vi "Proiect_senzori.vi"() -> ()   [LabVIEW 2024]
panel:
  out "Panou de control lumini":string
  in  "Lumina aprinsa garaj":bool
  in  "Lumina aprinsa debara":bool
  in  "Lumina aprinsa living":bool
  in  "Lumina aprinsa bucatarie":bool
  in  "Lumina aprinsa baie":bool
  in  "Lumina aprinsa hol":bool
  in  "Lumina aprinsa dormitor3":bool
  in  "Lumina aprinsa dormitor2":bool
  in  "Lumina aprinsa dormitor1":bool
  in  "Starea ventilatorului":bool
  in  "Min 2":dbl=18.0
  in  "Max 2":dbl=25.0
  out "?":string
  in  "Control umiditate":dbl(slide) scale=0.0..10.0
  in  "Temperatura":dbl(slide) scale=-20.0..60.0
  in  "a":bool
  out "Alarma":string
  out "Control geamuri":string
  out "?":string
  in  "Min":dbl=18.0
  in  "Max":dbl=25.0
  out "Securitate usa de la intrare":string
  in  "Introdu parola":dbl
  out "?":bool
  out "?":bool
  out "?":bool
  out "?":bool
  out "?":bool
  out "?":bool
  out "?":bool
  out "?":bool
  out "?":bool
  out "?":bool
  in  "Nivel luminã solarã":dbl(slide) scale=0.0..100.0
  out "Putere generata [W]":dbl(slide) scale=0.0..5000.0 scale format="%.2f"
  out "Control usi":string
  in  "Usa de la garaj":bool
  in  "Usa de la baie":bool
  in  "Usa de la dormitor 2":bool
  in  "Usa de la dormitor 3":bool
  in  "Usa de la dormitor 1":bool
  in  "Usa de la bucatarie":bool
  in  "Usa de la debara":bool
  in  "Usa de la living la garaj":bool
  in  "Usa de la living":bool
  in  "Usa de la intrare":bool
  in  "Senzor geam garaj":bool
  in  "Senzor de miscare  garaj":bool
  in  "Geam garaj":bool
  in  "Geam baie":bool
  in  "Geam dormitor3":bool
  in  "Geam dormitor2":bool
  in  "Geam dormitor1":bool
  in  "Geam debara":bool
  in  "Geam bucatarie 1":bool
  in  "Geam bucatarie 2":bool
  in  "Geam living 3":bool
  in  "Geam living 2":bool
  in  "Geam living 1":bool
  in  "Senzor de miscare  living":bool
  in  "Senzor geam living3":bool
  in  "Senzor geam living2":bool
  in  "Senzor geam living1":bool
  in  "Senzor geam dormitor3":bool
  in  "Senzor geam dormitor2":bool
  in  "Senzor geam baie":bool
  in  "Senzor geam dormitor1":bool
  in  "Senzor geam debara":bool
  in  "Senzor geam bucatarie2":bool
  in  "Senzor geam bucatarie1":bool
  in  "Senzor de miscare  baie":bool
  in  "Senzor de miscare dormitor3":bool
  in  "Senzor de miscare dormitor2":bool
  in  "Senzor de miscare dormitor1":bool
  in  "Senzor de miscare debara":bool
  in  "Senzor de miscare bucatarie":bool
  in  "Senzor de miscare hol":bool
  in  "stop":bool
  # "Planul casei inteligente"
  # "Bucatarie"
  # "Dormitor 1"
  # "Debara"
  # "Living"
  # "Hol"
  # "Garaj"
  # "Dormitor 3"
  # "Dormitor 2"
  # "Baie"
  # "Panou fotovoltaic"
  # "Reglare temperatura"
  # "Reglare umiditate"
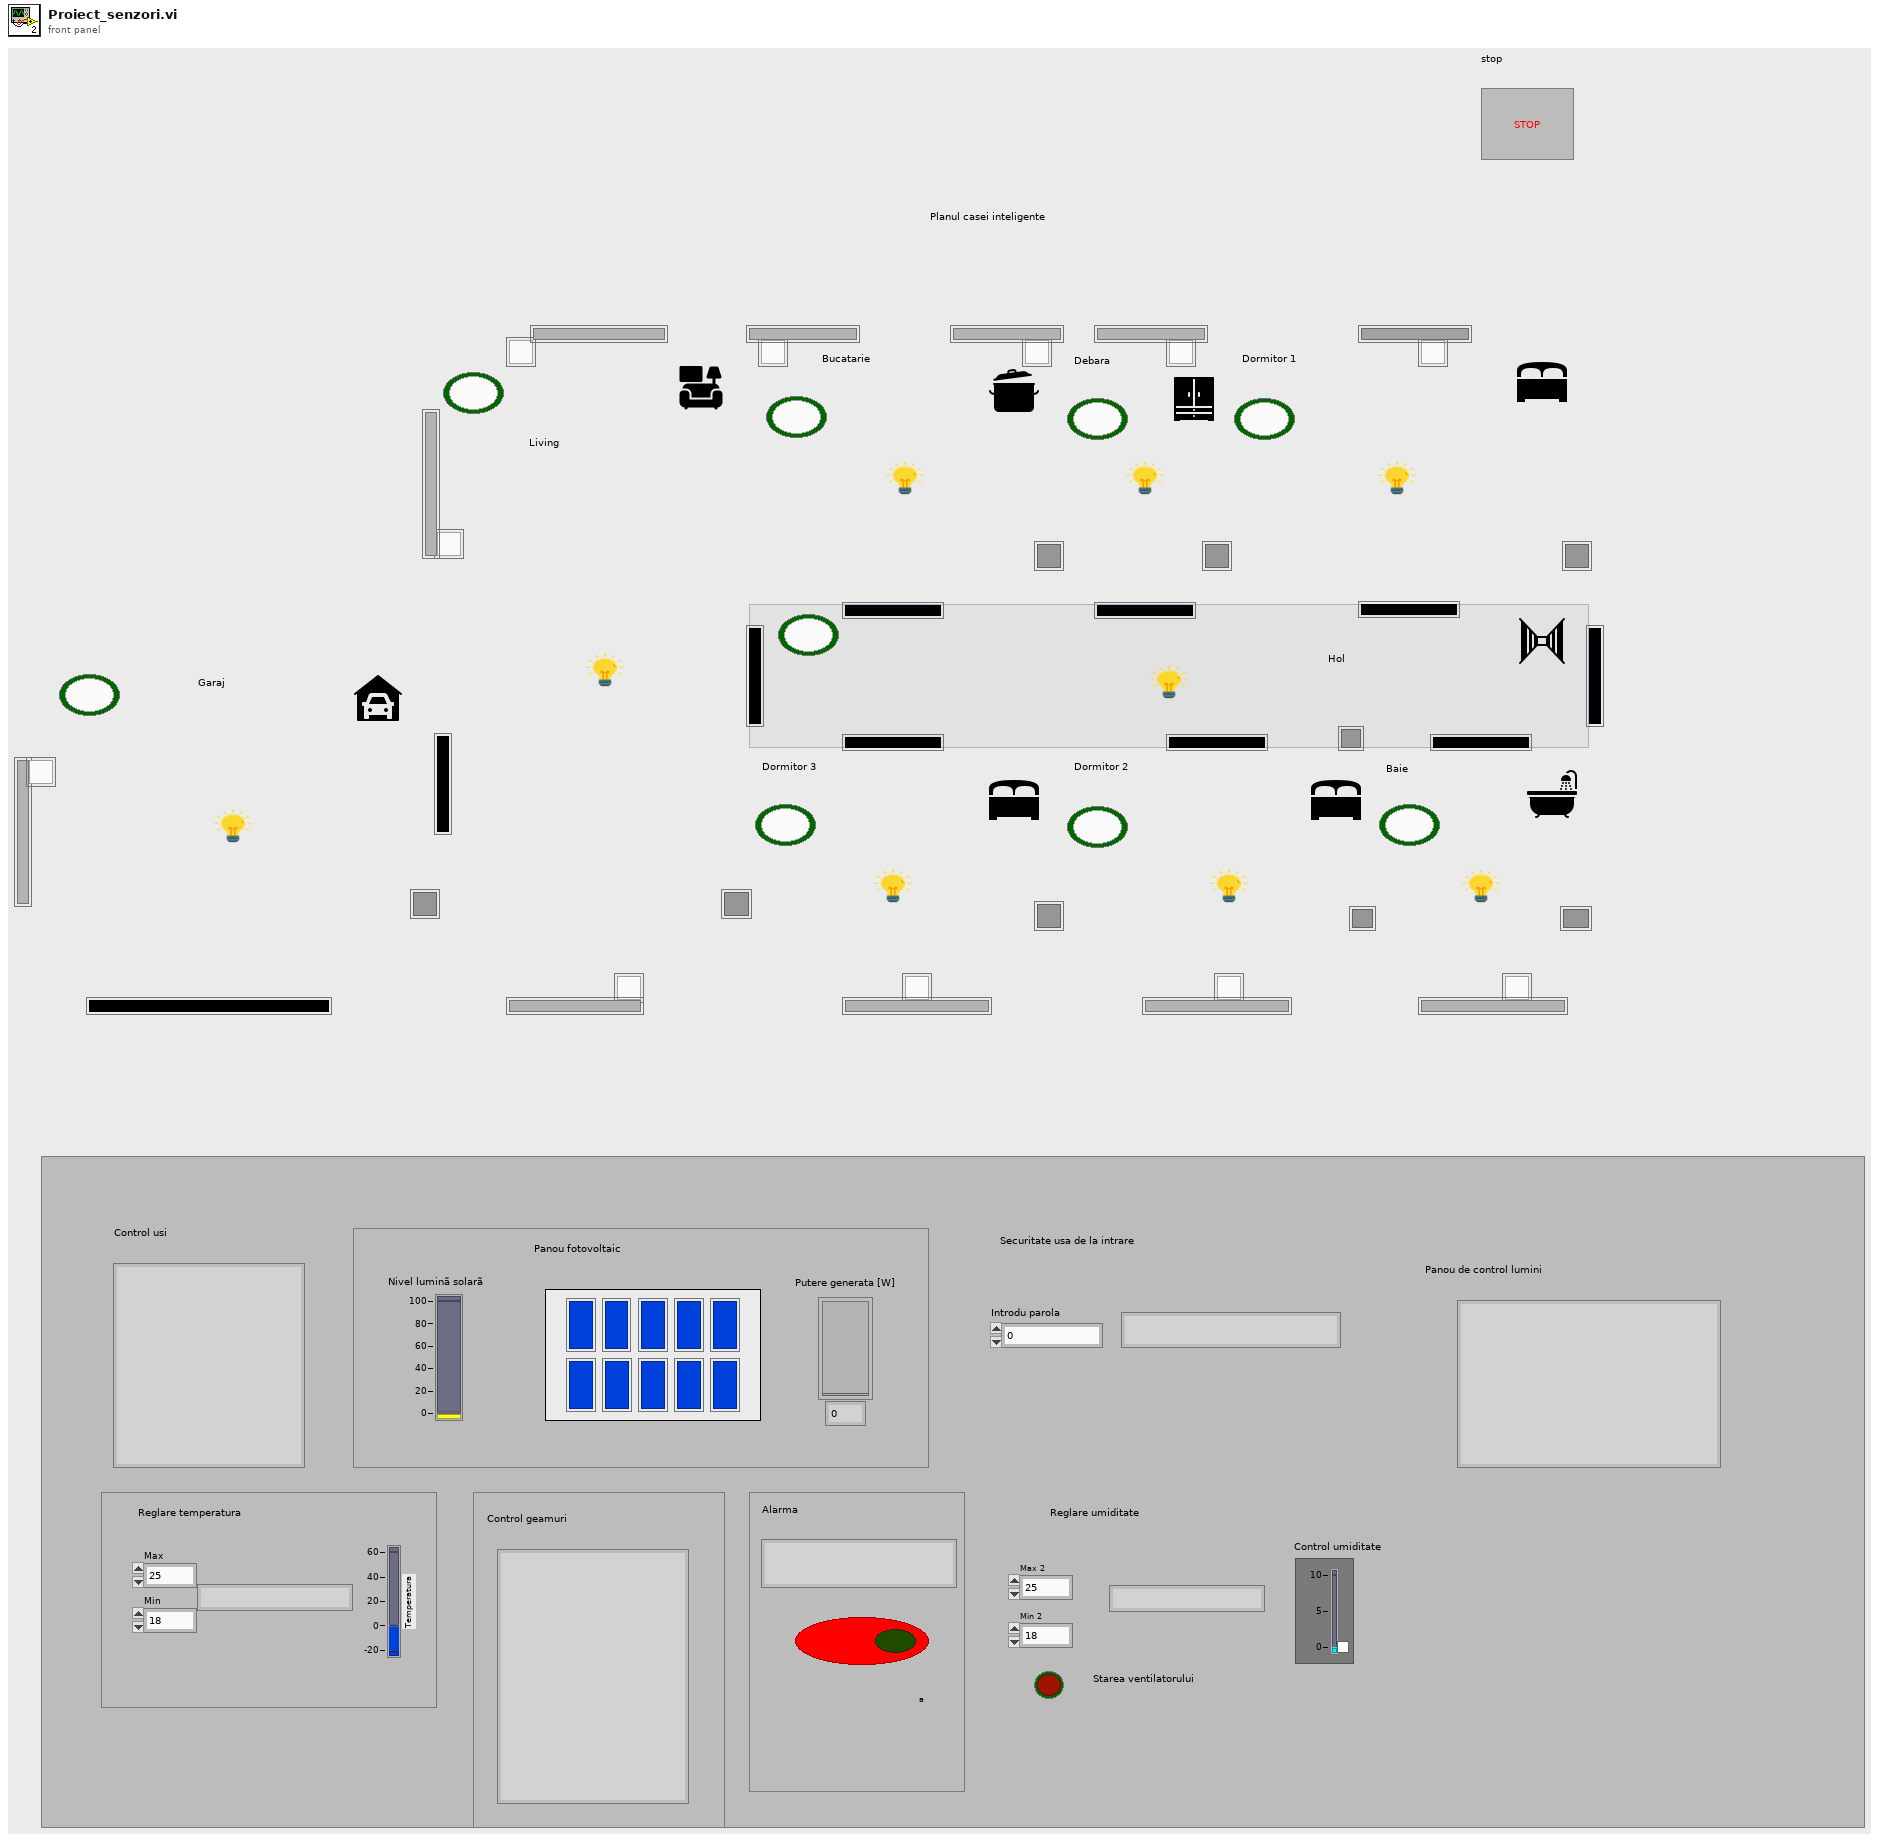
[diagram p1: front panel]
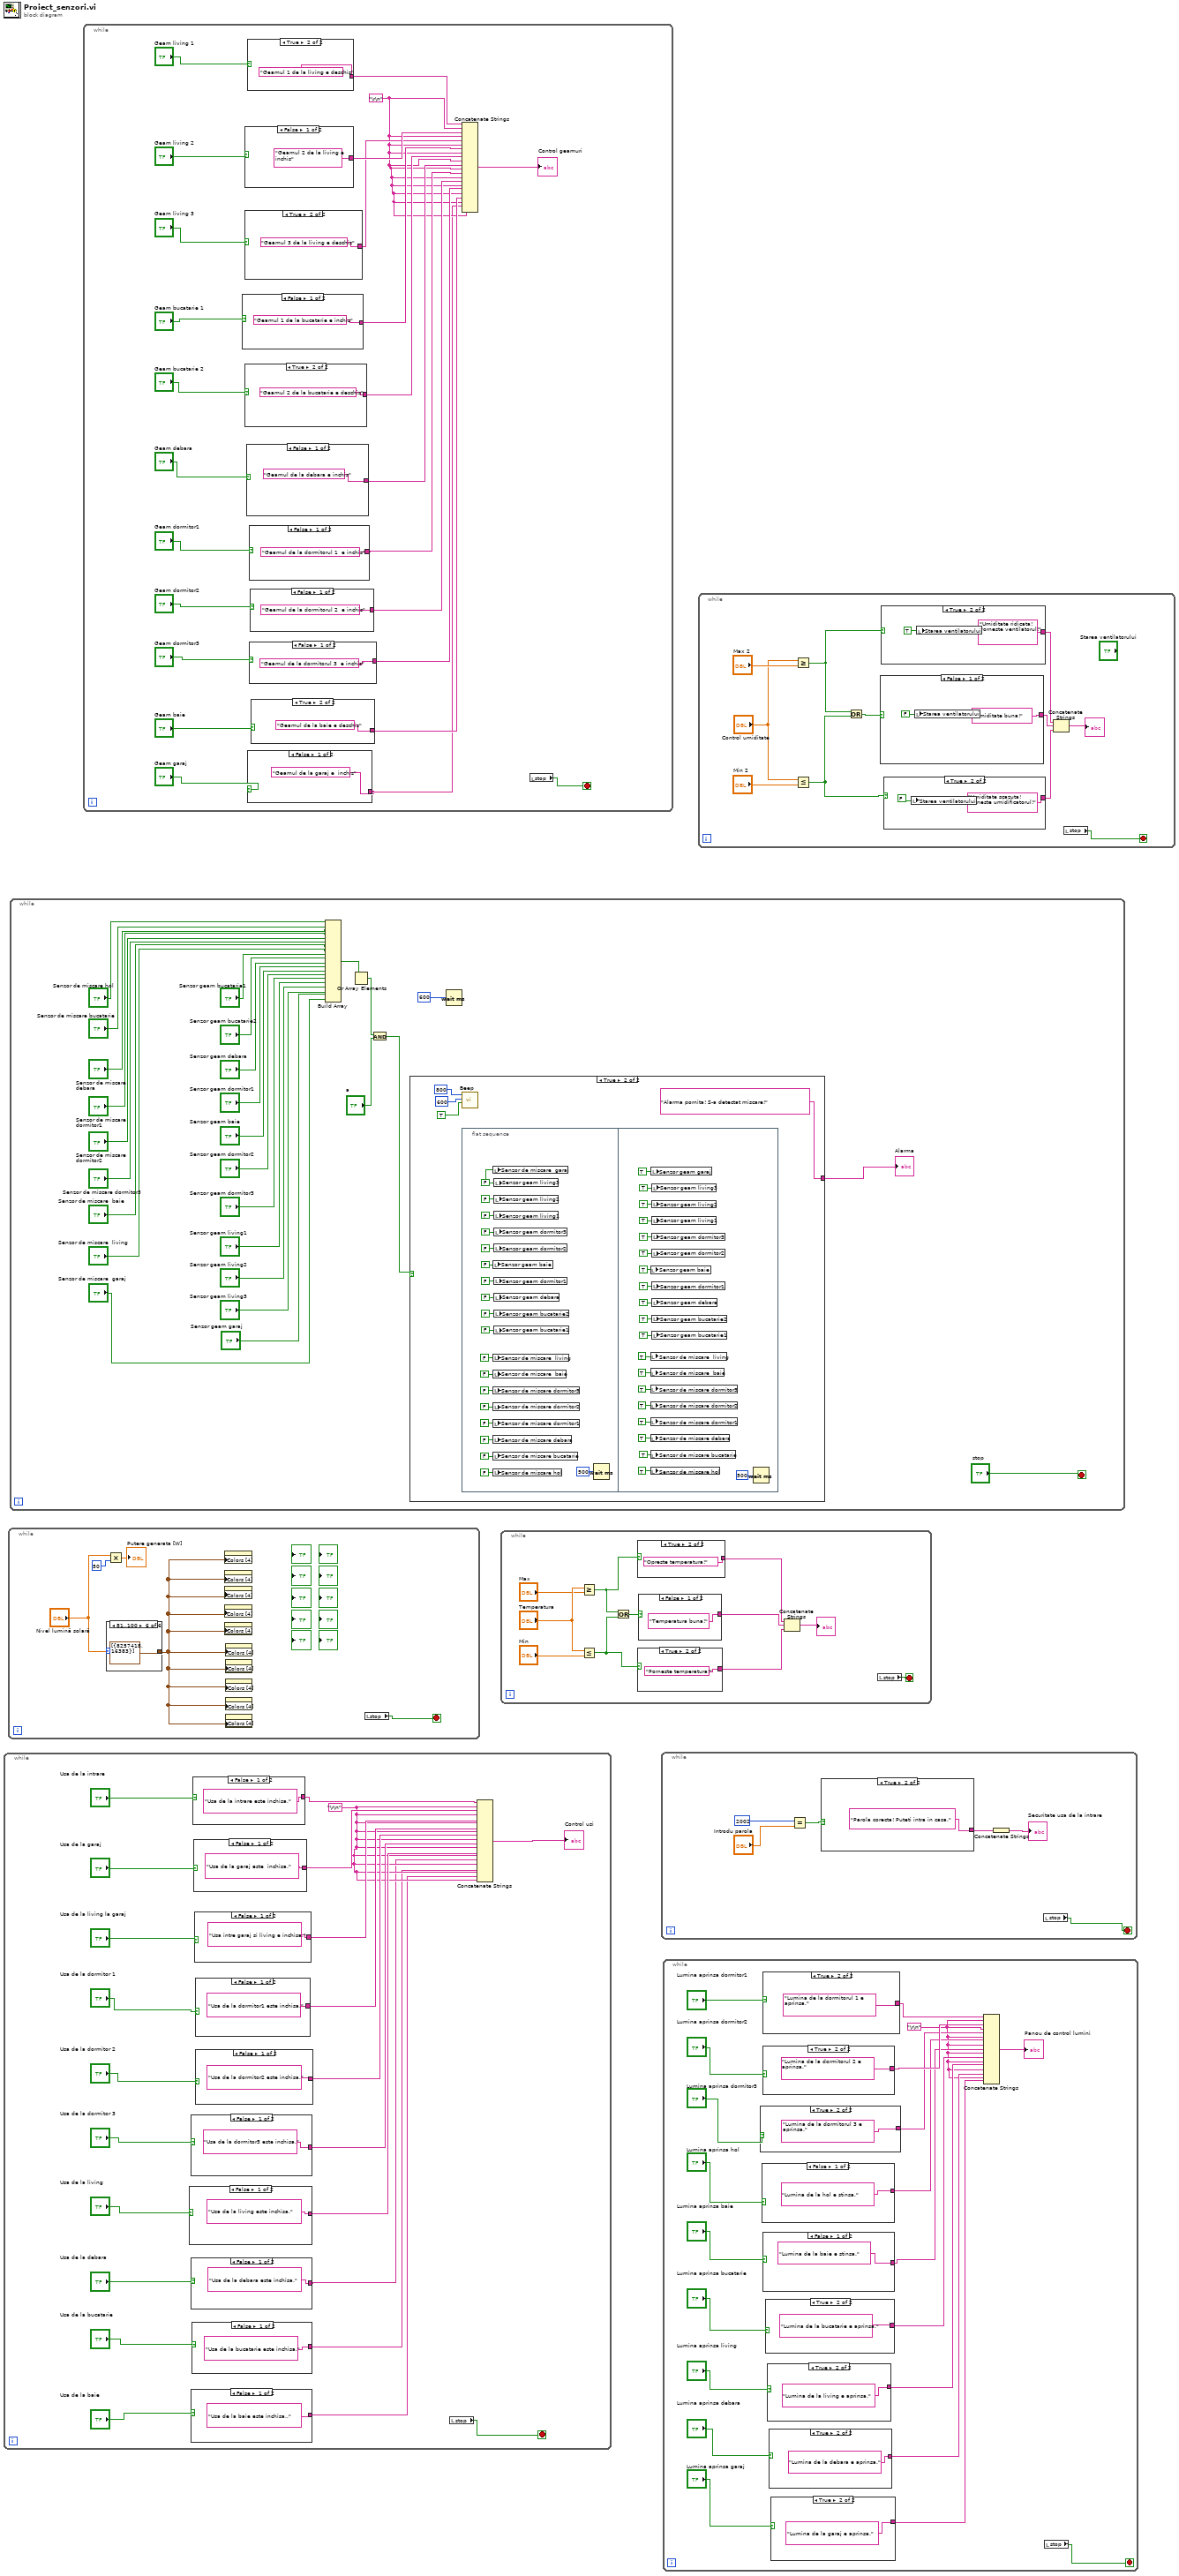
[diagram p0: block diagram]
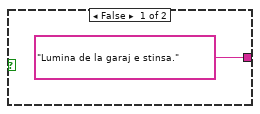
[diagram p2: hidden frame]
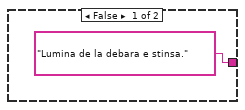
[diagram p3: hidden frame]
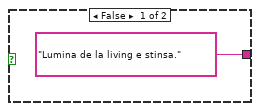
[diagram p4: hidden frame]
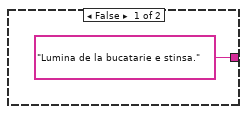
[diagram p5: hidden frame]
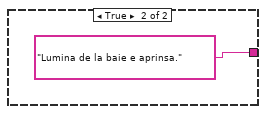
[diagram p6: hidden frame]
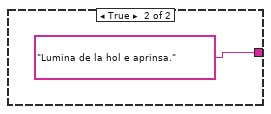
[diagram p7: hidden frame]
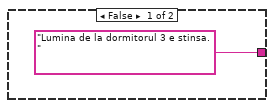
[diagram p8: hidden frame]
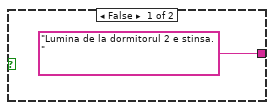
[diagram p9: hidden frame]
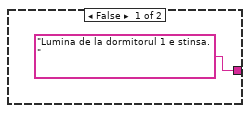
[diagram p10: hidden frame]
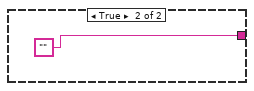
[diagram p11: hidden frame]
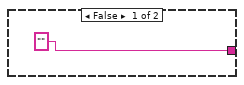
[diagram p12: hidden frame]
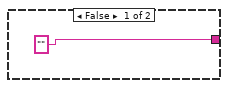
[diagram p13: hidden frame]
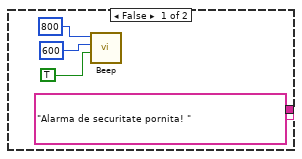
[diagram p14: hidden frame]
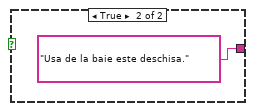
[diagram p15: hidden frame]
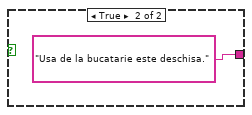
[diagram p16: hidden frame]
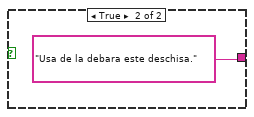
[diagram p17: hidden frame]
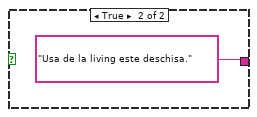
[diagram p18: hidden frame]
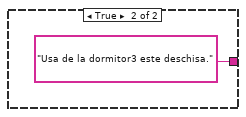
[diagram p19: hidden frame]
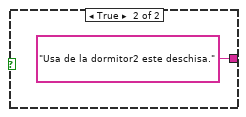
[diagram p20: hidden frame]
diagram:
  n1 = while {
    stop <- w1 stop-if-true
    w6 = "\r\n" ("End of Line Constant")
    n2 = case shown="False" "Usa de la living" {
      tunnel: ["Usa de la living este inchisa." "Usa de la living este deschisa."] -> w7
      frame False {
      }
      frame True {
      }
    }
    n3 = case shown="False" "Usa de la debara" {
      tunnel: ["Usa de la debara este inchisa." "Usa de la debara este deschisa."] -> w5
      frame False {
      }
      frame True {
      }
    }
    n4 = case shown="False" "Usa de la dormitor 3" {
      tunnel: ["Usa de la dormitor3 este inchisa." "Usa de la dormitor3 este deschisa."] -> w8
      frame False {
      }
      frame True {
      }
    }
    n5 = case shown="False" "Usa de la baie" {
      tunnel: ["Usa de la baie este inchisa.." "Usa de la baie este deschisa."] -> w3
      frame False {
      }
      frame True {
      }
    }
    n6 = case shown="False" "Usa de la bucatarie" {
      tunnel: ["Usa de la bucatarie este inchisa." "Usa de la bucatarie este deschisa."] -> w4
      frame False {
      }
      frame True {
      }
    }
    n7 = case shown="False" "Usa de la intrare" {
      tunnel: ["Usa de la intrare este inchisa," "Usa de la intrare este deschisa."] -> w13
      frame False {
      }
      frame True {
      }
    }
    n8 = case shown="False" "Usa de la garaj" {
      tunnel: ["Usa de la garaj este  inchisa." "Usa de la garaj este  deschisa."] -> w12
      frame False {
      }
      frame True {
      }
    }
    n9 = case shown="False" "Usa de la living la garaj" {
      tunnel: ["Usa intre garaj si living e inchisa." "Usa intre garaj si living e deschisa."] -> w11
      frame False {
      }
      frame True {
      }
    }
    n10 = case shown="False" "Usa de la dormitor 1" {
      tunnel: ["Usa de la dormitor1 este inchisa." "Usa de la dormitor1 este deschisa."] -> w10
      frame False {
      }
      frame True {
      }
    }
    n11 = case shown="False" "Usa de la dormitor 2" {
      tunnel: ["Usa de la dormitor2 este inchisa." "Usa de la dormitor2 este deschisa."] -> w9
      frame False {
      }
      frame True {
      }
    }
    n12 = local read "stop"() -> (w1:bool)
    n13 = Concatenate Strings(w13, w6, w12, w6, w11, w6, w10, w6, w9, w6, w8, w6, w7, w6, w5, w6, w4, w6, w3, w6) -> (→"Control usi":string)
  }
  n14 = while {
    stop <- w44 stop-if-true
    n15 = case shown="81..100" "Nivel luminã solarã" {
      tunnel: [cluster{u32, u32}[] [{16860, 16860}] ("Colors [4]") cluster{u32, u32}[] [{15366, 16383}] ("Colors [4]") cluster{u32, u32}[] [{42000, 16383}] ("Colors [4]") cluster{u32, u32}[] [{56598, 16383}] ("Colors [4]") cluster{u32, u32}[] [{2293560, 16383}] ("Colors [4]") cluster{u32, u32}[] [{8257418, 16383}] ("Colors [4]")] -> w45
      frame 0, Default {
      }
      frame 1..20 {
      }
      frame 21..40 {
      }
      frame 41..60 {
      }
      frame 61..80 {
      }
      frame 81..100 {
      }
    }
    n16 = Multiply(x="Nivel luminã solarã", y=50) -> (x*y=→"Putere generata [W]":dbl)
    n17 = property class="Bool (strict)"("Colors [4]"=w45) -> ()  [unwired: 2 in, 2 out]
    n18 = property class="Bool (strict)"("Colors [4]"=w45) -> ()  [unwired: 2 in, 2 out]
    n19 = property class="Bool (strict)"("Colors [4]"=w45) -> ()  [unwired: 2 in, 2 out]
    n20 = property class="Bool (strict)"("Colors [4]"=w45) -> ()  [unwired: 2 in, 2 out]
    n21 = property class="Bool (strict)"("Colors [4]"=w45) -> ()  [unwired: 2 in, 2 out]
    n22 = property class="Bool (strict)"("Colors [4]"=w45) -> ()  [unwired: 2 in, 2 out]
    n23 = property class="Bool (strict)"("Colors [4]"=w45) -> ()  [unwired: 2 in, 2 out]
    n24 = property class="Bool (strict)"("Colors [4]"=w45) -> ()  [unwired: 2 in, 2 out]
    n25 = property class="Bool (strict)"("Colors [4]"=w45) -> ()  [unwired: 2 in, 2 out]
    n26 = property class="Bool (strict)"("Colors [4]"=w45) -> ()  [unwired: 2 in, 2 out]
    n27 = local read "stop"() -> (w44:bool)
  }
  n28 = while {
    stop <- "stop" stop-if-true
    n29 = Build Array "Build Array"("Senzor de miscare hol", "Senzor de miscare bucatarie", "Senzor de miscare debara", "Senzor de miscare dormitor1", "Senzor de miscare dormitor2", "Senzor de miscare dormitor3", "Senzor de miscare  baie", "Senzor de miscare  living", "Senzor geam bucatarie1", "Senzor geam bucatarie2", "Senzor geam debara", "Senzor geam dormitor1", "Senzor geam baie", "Senzor geam dormitor2", "Senzor geam dormitor3", "Senzor geam living1", "Senzor geam living2", "Senzor geam living3", "Senzor geam garaj", "Senzor de miscare  garaj") -> (w80:bool[])
    n30 = Or Array Elements(Boolean array=w80) -> (logical OR=w58:bool)
    n31 = And(x=w58, y="a") -> (x .and. y?=w56:bool)
    n32 = case shown="True" w56 {
      tunnel: ["Alarma oprita! Nu avem niciun pericol. " "Alarma pornita! S-a detectat miscare!"] -> w61
      frame False {
      }
      frame True {
        n33 = call <vilib>:"Beep.vi"("use system alert? (T)"=TRUE, "duration (msec)"=600, "frequency (Hz)"=800) -> ()  [unwired: 9 in]
        n34 = flat-sequence {
          frame #0 {
            w87 = FALSE ("Senzor geam living3")
            n35 = local write "Senzor de miscare  garaj"(w87) -> ()
            n36 = local write "Senzor geam baie"(FALSE ("Senzor geam baie")) -> ()
            n37 = local write "Senzor de miscare  living"(FALSE ("Senzor de miscare  living")) -> ()
            n38 = local write "Senzor de miscare  baie"(FALSE ("Senzor de miscare  baie")) -> ()
            n39 = local write "Senzor de miscare dormitor3"(FALSE ("Senzor de miscare dormitor3")) -> ()
            n40 = local write "Senzor de miscare dormitor2"(FALSE ("Senzor de miscare dormitor2")) -> ()
            n41 = local write "Senzor de miscare dormitor1"(FALSE ("Senzor de miscare dormitor1")) -> ()
            n42 = local write "Senzor de miscare debara"(FALSE ("Senzor de miscare debara")) -> ()
            n43 = local write "Senzor de miscare bucatarie"(FALSE ("Senzor de miscare bucatarie")) -> ()
            n44 = local write "Senzor de miscare hol"(FALSE ("Senzor de miscare hol")) -> ()
            n45 = local write "Senzor geam living3"(w87) -> ()
            n46 = local write "Senzor geam living2"(FALSE ("Senzor geam living2")) -> ()
            n47 = local write "Senzor geam living1"(FALSE ("Senzor geam living1")) -> ()
            n48 = local write "Senzor geam dormitor3"(FALSE ("Senzor geam dormitor3")) -> ()
            n49 = local write "Senzor geam dormitor2"(FALSE ("Senzor geam dormitor2")) -> ()
            n50 = local write "Senzor geam dormitor1"(FALSE ("Senzor geam dormitor1")) -> ()
            n51 = local write "Senzor geam debara"(FALSE ("Senzor geam debara")) -> ()
            n52 = local write "Senzor geam bucatarie2"(FALSE ("Senzor geam bucatarie2")) -> ()
            n53 = local write "Senzor geam bucatarie1"(FALSE ("Senzor geam bucatarie1")) -> ()
            n54 = Wait (ms)(milliseconds to wait=u32 500) -> ()  [unwired: 1 out]
          }
          frame #1 {
            n55 = local write "Senzor geam baie"(TRUE ("Senzor geam baie")) -> ()
            n56 = local write "Senzor de miscare  living"(TRUE ("Senzor de miscare  living")) -> ()
            n57 = local write "Senzor de miscare  baie"(TRUE ("Senzor de miscare  baie")) -> ()
            n58 = local write "Senzor de miscare dormitor3"(TRUE ("Senzor de miscare dormitor3")) -> ()
            n59 = local write "Senzor de miscare dormitor2"(TRUE ("Senzor de miscare dormitor2")) -> ()
            n60 = local write "Senzor de miscare dormitor1"(TRUE ("Senzor de miscare dormitor1")) -> ()
            n61 = local write "Senzor de miscare debara"(TRUE ("Senzor de miscare debara")) -> ()
            n62 = local write "Senzor de miscare bucatarie"(TRUE ("Senzor de miscare bucatarie")) -> ()
            n63 = local write "Senzor de miscare hol"(TRUE ("Senzor de miscare hol")) -> ()
            n64 = local write "Senzor geam garaj"(TRUE ("Senzor geam garaj")) -> ()
            n65 = local write "Senzor geam living3"(TRUE ("Senzor geam living3")) -> ()
            n66 = local write "Senzor geam living2"(TRUE ("Senzor geam living2")) -> ()
            n67 = local write "Senzor geam living1"(TRUE ("Senzor geam living1")) -> ()
            n68 = local write "Senzor geam dormitor3"(TRUE ("Senzor geam dormitor3")) -> ()
            n69 = local write "Senzor geam dormitor2"(TRUE ("Senzor geam dormitor2")) -> ()
            n70 = local write "Senzor geam dormitor1"(TRUE ("Senzor geam dormitor1")) -> ()
            n71 = local write "Senzor geam debara"(TRUE ("Senzor geam debara")) -> ()
            n72 = local write "Senzor geam bucatarie2"(TRUE ("Senzor geam bucatarie2")) -> ()
            n73 = local write "Senzor geam bucatarie1"(TRUE ("Senzor geam bucatarie1")) -> ()
            n74 = Wait (ms)(milliseconds to wait=u32 500) -> ()  [unwired: 1 out]
          }
        }
      }
    }
    "Alarma" <- w61
    n75 = Wait (ms)(milliseconds to wait=600) -> ()  [unwired: 1 out]
  }
  n76 = while {
    stop <- w126 stop-if-true
    w128 = "\r\n" ("End of Line Constant")
    n77 = case shown="False" "Geam bucatarie 1" {
      tunnel: ["Geamul 1 de la bucatarie e inchis" "Geamul 1 de la bucatarie e deschis"] -> w143
      frame False {
      }
      frame True {
      }
    }
    n78 = case shown="False" "Geam living 2" {
      tunnel: ["Geamul 2 de la living e inchis" "Geamul 2 de la living e deschis"] -> w145
      frame False {
      }
      frame True {
      }
    }
    n79 = case shown="True" "Geam living 3" {
      tunnel: ["Geamul 2 de la living e inchis" "Geamul 3 de la living e deschis"] -> w144
      frame False {
      }
      frame True {
      }
    }
    n80 = case shown="True" "Geam bucatarie 2" {
      tunnel: ["Geamul 2 de la bucatarie e inchis" "Geamul 2 de la bucatarie e deschis"] -> w140
      frame False {
      }
      frame True {
      }
    }
    n81 = case shown="False" "Geam debara" {
      tunnel: ["Geamul de la debara e inchis" "Geamul de la debara e deschis"] -> w139
      frame False {
      }
      frame True {
      }
    }
    n82 = case shown="True" "Geam living 1" {
      tunnel: ["Geamul 1 de la living e inchis" "Geamul 1 de la living e deschis"] -> w147
      frame False {
      }
      frame True {
      }
    }
    n83 = case shown="False" "Geam garaj" {
      tunnel: ["Geamul de la garaj e  inchis" "Geamul de la garaj e deschis"] -> w127
      frame False {
      }
      frame True {
      }
    }
    n84 = case shown="False" "Geam dormitor1" {
      tunnel: ["Geamul de la dormitorul 1  e inchis" "Geamul de la dormitorul 1 e deschis"] -> w136
      frame False {
      }
      frame True {
      }
    }
    n85 = case shown="False" "Geam dormitor3" {
      tunnel: ["Geamul de la dormitorul 3  e inchis" "Geamul de la dormitorul 3 e deschis"] -> w132
      frame False {
      }
      frame True {
      }
    }
    n86 = case shown="False" "Geam dormitor2" {
      tunnel: ["Geamul de la dormitorul 2  e inchis" "Geamul de la dormitorul 2 e deschis"] -> w133
      frame False {
      }
      frame True {
      }
    }
    n87 = case shown="True" "Geam baie" {
      tunnel: ["Geamul de la baie e inchis" "Geamul de la baie e deschis"] -> w131
      frame False {
      }
      frame True {
      }
    }
    n88 = Concatenate Strings(w147, w128, w145, w128, w144, w128, w143, w128, w140, w128, w139, w128, w136, w128, w133, w128, w132, w128, w131, w128, w127, w128) -> (→"Control geamuri":string)
    n89 = local read "stop"() -> (w126:bool)
  }
  n90 = while {
    stop <- w173 stop-if-true
    n91 = Greater Or Equal?(x="Temperatura", y="Max") -> (x >= y?=w177:bool)
    n92 = Less Or Equal?(x="Temperatura", y="Min") -> (x <= y?=w176:bool)
    n93 = Or(x=w177, y=w176) -> (x .or. y?=w175:bool)
    n94 = case shown="True" w177 {
      tunnel: ["" "Opreste temperatura!"] -> w179
      frame False {
      }
      frame True {
      }
    }
    n95 = case shown="True" w176 {
      tunnel: ["" "Porneste temperatura!"] -> w178
      frame False {
      }
      frame True {
      }
    }
    n96 = case shown="False" w175 {
      tunnel: ["Temperatura buna!" ""] -> w174
      frame False {
      }
      frame True {
      }
    }
    n97 = Concatenate Strings(w179, w174, w178) -> (→"?":string)
    n98 = local read "stop"() -> (w173:bool)
  }
  n99 = while {
    stop <- w190 stop-if-true
    n100 = Equal?(x=2002, y="Introdu parola") -> (x = y?=w193:bool)
    n101 = case shown="True" w193 {
      tunnel: ["Alarma de securitate pornita! " "Parola corecta! Puteti intra in casa."] -> w192
      frame False {
        n102 = call <vilib>:"Beep.vi"("use system alert? (T)"=TRUE, "duration (msec)"=600, "frequency (Hz)"=800) -> ()  [unwired: 9 in]
      }
      frame True {
      }
    }
    n103 = Concatenate Strings(w192) -> (→"Securitate usa de la intrare":string)
    n104 = local read "stop"() -> (w190:bool)
  }
  n105 = while {
    stop <- w201 stop-if-true
    w203 = "\r\n" ("End of Line Constant")
    n106 = case shown="True" "Lumina aprinsa dormitor3" {
      tunnel: ["Lumina de la dormitorul 3 e stinsa." "Lumina de la dormitorul 3 e aprinsa."] -> w209
      frame False {
      }
      frame True {
      }
    }
    n107 = case shown="False" "Lumina aprinsa hol" {
      tunnel: ["Lumina de la hol e stinsa." "Lumina de la hol e aprinsa."] -> w208
      frame False {
      }
      frame True {
      }
    }
    n108 = case shown="True" "Lumina aprinsa dormitor2" {
      tunnel: ["Lumina de la dormitorul 2 e stinsa." "Lumina de la dormitorul 2 e aprinsa."] -> w210
      frame False {
      }
      frame True {
      }
    }
    n109 = case shown="False" "Lumina aprinsa baie" {
      tunnel: ["Lumina de la baie e stinsa." "Lumina de la baie e aprinsa."] -> w207
      frame False {
      }
      frame True {
      }
    }
    n110 = case shown="True" "Lumina aprinsa dormitor1" {
      tunnel: ["Lumina de la dormitorul 1 e stinsa." "Lumina de la dormitorul 1 e aprinsa."] -> w211
      frame False {
      }
      frame True {
      }
    }
    n111 = case shown="True" "Lumina aprinsa bucatarie" {
      tunnel: ["Lumina de la bucatarie e stinsa." "Lumina de la bucatarie e aprinsa."] -> w206
      frame False {
      }
      frame True {
      }
    }
    n112 = case shown="True" "Lumina aprinsa living" {
      tunnel: ["Lumina de la living e stinsa." "Lumina de la living e aprinsa."] -> w205
      frame False {
      }
      frame True {
      }
    }
    n113 = case shown="True" "Lumina aprinsa debara" {
      tunnel: ["Lumina de la debara e stinsa." "Lumina de la debara e aprinsa."] -> w204
      frame False {
      }
      frame True {
      }
    }
    n114 = case shown="True" "Lumina aprinsa garaj" {
      tunnel: ["Lumina de la garaj e stinsa." "Lumina de la garaj e aprinsa."] -> w202
      frame False {
      }
      frame True {
      }
    }
    n115 = Concatenate Strings(w211, w203, w210, w203, w209, w203, w208, w203, w207, w203, w206, w203, w205, w203, w204, w203, w202) -> (→"Panou de control lumini":string)
    n116 = local read "stop"() -> (w201:bool)
  }
  n117 = while {
    stop <- w250 stop-if-true
    n118 = Greater Or Equal?(x="Control umiditate", y="Max 2") -> (x >= y?=w244:bool)
    n119 = Less Or Equal?(x="Control umiditate", y="Min 2") -> (x <= y?=w243:bool)
    n120 = Or(x=w244, y=w243) -> (x .or. y?=w242:bool)
    n121 = case shown="False" w242 {
      tunnel: ["Umiditate buna!" ""] -> w241
      frame False {
        n122 = local write "Starea ventilatorului"(FALSE ("Porneste ventilatorul")) -> ()
      }
      frame True {
      }
    }
    n123 = case shown="True" w244 {
      tunnel: ["" "Umiditate ridicata! Porneste ventilatorul!"] -> w246
      frame False {
      }
      frame True {
        n124 = local write "Starea ventilatorului"(TRUE ("Porneste ventilatorul")) -> ()
      }
    }
    n125 = case shown="True" w243 {
      tunnel: ["" "Umiditate scazuta! Porneste umidificatorul!"] -> w245
      frame False {
      }
      frame True {
        n126 = local write "Starea ventilatorului"(FALSE ("Porneste ventilatorul")) -> ()
      }
    }
    n127 = Concatenate Strings(w246, w241, w245) -> (→"?":string)
    n128 = local read "stop"() -> (w250:bool)
  }
